vi "Equals.vi"(1 "comparable 2":refnum<class "Equal Comparable.lvclass">, 2 "comparable 1":refnum<class "Equal Comparable.lvclass">) -> (0 "less?":bool)   [LabVIEW 2020, in "Equal Comparable.lvclass"]
doc: "Returns whether <b>Comparable 1</b> is less than, equal to, or greater than <b>Comparable 2</b>."
uses:
  <vilib>/Comparison/Equal/Equal Comparable/Equal Comparable.lvclass
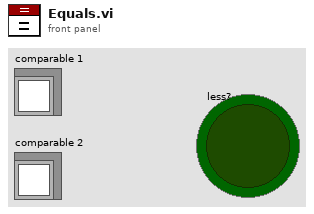
[diagram p1: front panel]
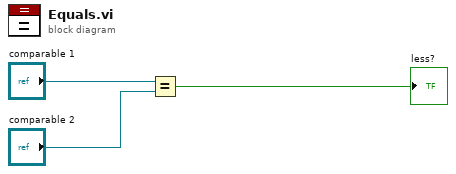
[diagram p0: block diagram]
diagram:
  n1 = Equal?(x="comparable 1", y="comparable 2") -> (x = y?=→"less?":bool)
